vi "DHT.vi"(10 "Error In":errorcluster, 11 "Serial Port":refnum<visa-resource-name>="N/A") -> (1 "Error Out":errorcluster, 2 "Temp ^C":u8(knob) scale=0.0..50.0, 3 "Humidity %":u8(knob) scale=0.0..100.0, 9 "LINX Resource":T1)   [LabVIEW 2020]
uses:
  <vilib>/MakerHub/LINX/Private/Type Defs/LINX Ref.ctl
  <vilib>/MakerHub/LINX/Private/Type Defs/Platform.ctl
  <vilib>/MakerHub/LINX/Private/Type Defs/Interface.ctl
  <vilib>/MakerHub/LINX/Private/Device/Type Defs/LINX Device Config.ctl
  <vilib>/MakerHub/LINX/Private/Device/Type Defs/TCP Config.ctl
  <vilib>/MakerHub/LINX/Private/Device/Type Defs/Channels.ctl
  <vilib>/MakerHub/LINX/Public/Utilities/Open Serial.vi
  <vilib>/MakerHub/LINX/LMH-LINX.lvlib
  <vilib>/MakerHub/LINX/Private/Device/Device.lvlib
panel:
  in  "?":bool
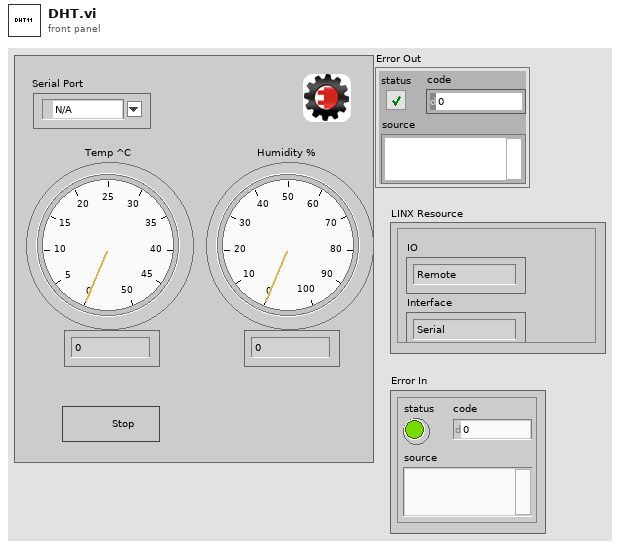
[diagram p1: front panel]
types:
  T1 = typedef "LMH-LINX.lvlib/LINX Ref.ctl" = cluster{"IO":T2, "Interface":T3, "LINX Device Config":T4}
  T2 = typedef "LMH-LINX.lvlib/Platform.ctl" = enum16{"Remote", "Local"}
  T3 = typedef "LMH-LINX.lvlib/Interface.ctl" = enum16{"Serial", "TCP"}
  T4 = typedef "LMH-LINX.lvlib/Device.lvlib/LINX Device Config.ctl" = cluster{"Interface":T3, "COM Port":refnum<visa-resource-name>, "TCP Configuration":T5, "Device Family":u8, "Device ID":u8, "Device Name":string, "TCP Ref":refnum<k5>, "Channels":T6}
  T5 = typedef "LMH-LINX.lvlib/Device.lvlib/TCP Config.ctl" = cluster{"IP Address":string, "Port":u16}
  T6 = typedef "LMH-LINX.lvlib/Channels.ctl" = cluster{"DI":u8[], "DO":u8[], "AI":u8[], "AO":u8[], "PWM":u8[], "QE":u8[], "UART":u8[], "I2C 2":u8[], "SPI":u8[], "CAN":u8[], "Servo":u8[], "AI Ref (V)":dbl, "AI Resolution (Bits)":u8, "AO Ref (V)":dbl, "AO Resolution (Bits)":u8}
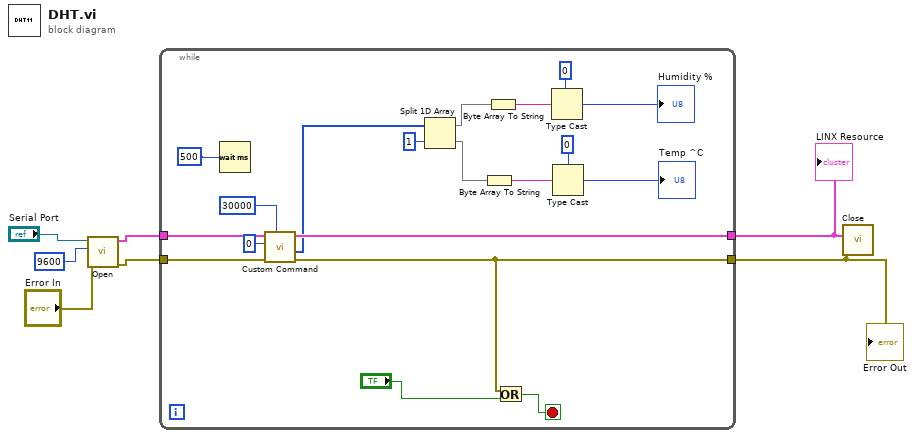
[diagram p0: block diagram]
diagram:
  n1 = call-poly <vilib>:"Open.vi"("Error In"="Error In", "Baud Rate Override"=u32 9600, "Serial Port"="Serial Port") -> ("Error Out"=w6:errorcluster, "LINX Resource"=w7:T1)  [unwired: 6 in, 1 out]
  n2 = while {
    tunnel: w7 -> [w26]
    tunnel: w6 -> [w25]
    tunnel: [w24] -> w5
    tunnel: [w22] -> w4
    stop <- w21 stop-if-true
    n3 = Wait (ms)(milliseconds to wait=u32 500) -> ()  [unwired: 1 out]
    n4 = call <vilib>:"Custom Command.vi"("Timeout (100 ms)"=30000, "Error In"=w25, "Custom Command Number"=u16 0, "LINX Resource"=w26) -> ("Error Out"=w22:errorcluster, "Response"=w18:u8[], "LINX Resource"=w24:T1)  [unwired: 4 in, 1 out]
    n5 = Split 1D Array(array=w18, index=1) -> (first subarray=w16:u8[], second subarray=w15:u8[])
    n6 = Byte Array To String(unsigned byte array=w15) -> (string=w11:string)
    n7 = Byte Array To String(unsigned byte array=w16) -> (string=w13:string)
    n8 = Or(x=w22, y="?") -> (x .or. y?=w21:bool)
    n9 = Type Cast(type=u8 0, x=w13) -> (*(type *) &x=→"Humidity %":u8)
    n10 = Type Cast(type=u8 0, x=w11) -> (*(type *) &x=→"Temp ^C":u8)
  }
  "Error Out" <- w4
  "LINX Resource" <- w5
  n11 = call <vilib>:"Close.vi"("Error In"=w4, "LINX Resource"=w5) -> ()  [unwired: 9 in, 1 out]
